vi "SettingParameter_Excel_to_VI.vi"() -> ()   [LabVIEW 2014]
uses:
  <vilib>/Utility/file.llb/Read From Spreadsheet File (string).vi
panel:
  out "subarray":string[](array[string])
  in  "Name 12":dbl
  in  "Name 11":dbl
  in  "Name 10":dbl
  in  "Name 9":dbl
  in  "Name 8":dbl
  in  "Name 7":dbl
  in  "Name 6":dbl
  in  "Name 5":dbl
  in  "Name 4":dbl
  in  "Name 3":dbl
  in  "Name 2":dbl
  in  "Name 1":dbl
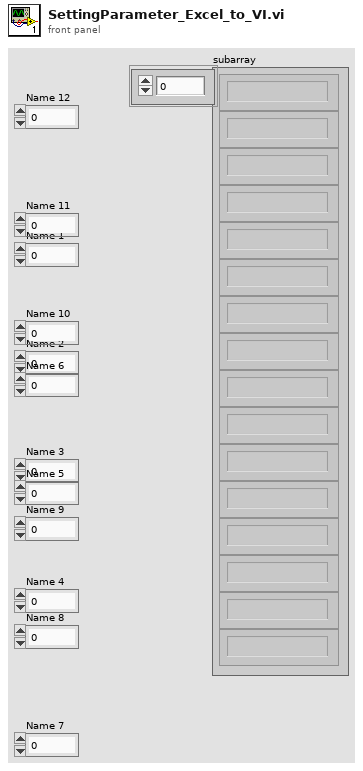
[diagram p1: front panel]
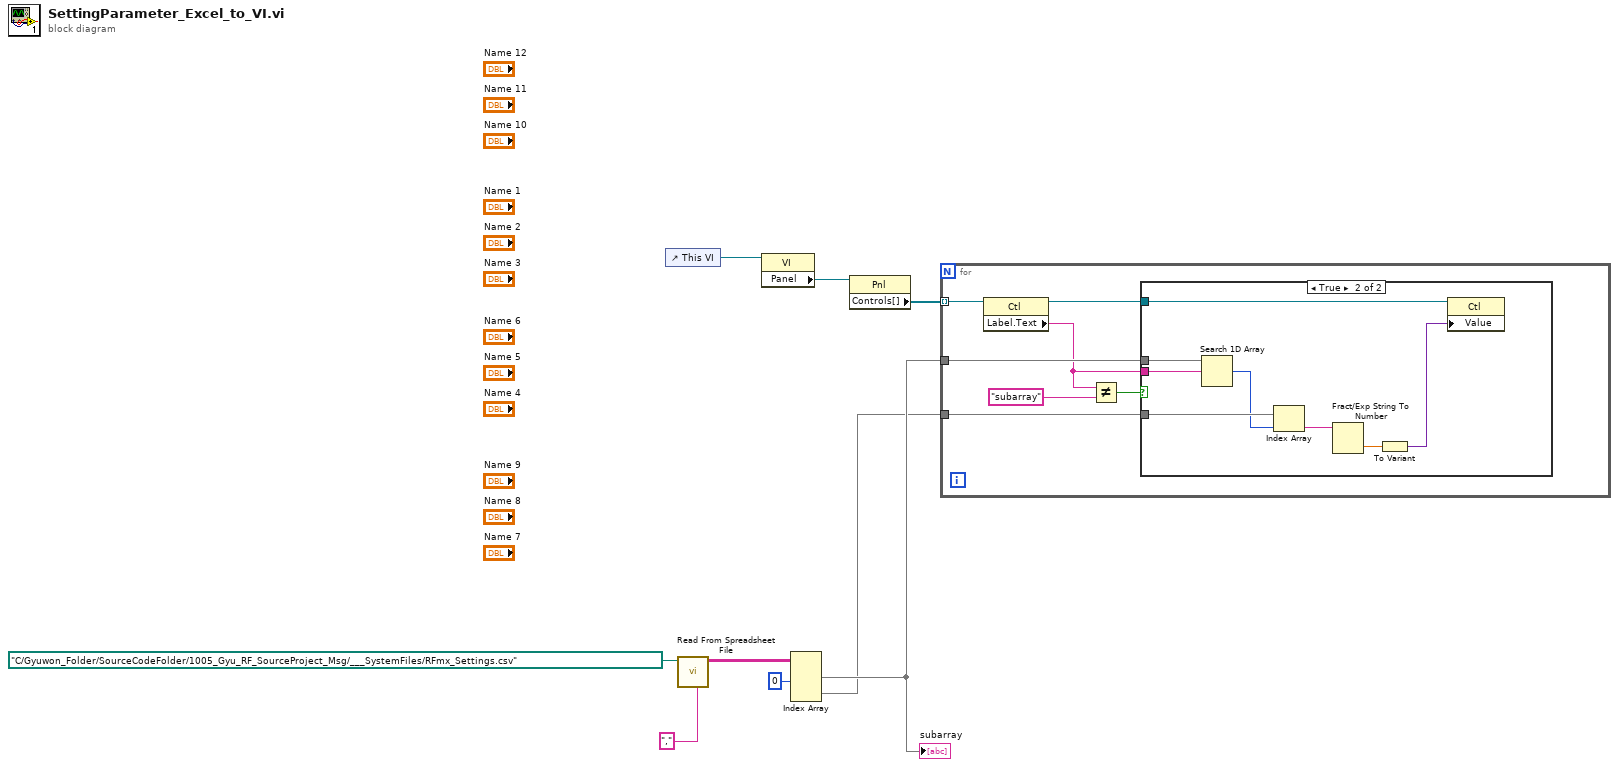
[diagram p0: block diagram]
diagram:
  n1 = control-ref of="This VI"() -> (w9:refnum<vi>)
  n2 = call-poly <vilib>:"Read From Spreadsheet File.vi"("delimiter (\\t)"="," ("delimiter (\\t)"), "file path (dialog if empty)"=path "C:/Gyuwon_Folder/SourceCodeFolder/1005_Gyu_RF_SourceProject_Msg/___SystemFiles/RFmx_Settings.csv") -> ("all rows"=w5:string[][])  [unwired: 5 in, 4 out]
  n3 = property class="VI"(reference=w9) -> ("Panel"=w8:refnum<vi>)  [unwired: 1 in, 2 out]
  n4 = Index Array(array=w5, index (col) #1=0 ("disabled index (col)")) -> (element #1=w2:string[], element #2=w1:string[])  [unwired: 3 in]
  "subarray" <- w2
  n5 = property class="Pnl"(reference=w8) -> ("Controls[]"=w7:refnum<vi>[])  [unwired: 1 in, 2 out]
  n6 = for {
    tunnel: w7 -> [w16] mode=indexing
    tunnel: w2 -> [w15]
    tunnel: w1 -> [w14]
    n7 = property class="Ctl"(reference=w16) -> (reference out=w13:refnum<vi>, "Label.Text"=w11:string)  [unwired: 1 in, 1 out]
    n8 = Not Equal?(x=w11, y="subarray") -> (x != y?=w12:bool)
    n9 = case shown="True" w12 {
      tunnel: w15 -> [_ w24]
      tunnel: w11 -> [_ w23]
      tunnel: w14 -> [_ w22]
      tunnel: w13 -> [_ w18]
      frame False {
      }
      frame True {
        n10 = Search 1D Array(1D array=w24, element=w23) -> (index of element=w21:i32)  [unwired: 1 in]
        n11 = Index Array(array=w22, index=w21) -> (element=w20:string)
        n12 = Fract/Exp String To Number(string=w20) -> (number=w19:dbl)  [unwired: 3 in, 1 out]
        n13 = To Variant(anything=w19) -> (Variant=w17:variant)
        n14 = property class="Ctl"(reference=w18, "Value"=w17) -> ()  [unwired: 1 in, 2 out]
      }
    }
  }
